vi "TagDB Refmgr-Parse Rules.vi"(0 "DB Ref":T3, 5 "Rules":T1[](array[typedef]), 11 "error in (no error)":errorcluster) -> (4 "DB Ref (dup)":T3, 6 "StateNames":string[](array[string]), 10 "RulesMap":variant[](array[variant]), 15 "error out":errorcluster)   [LabVIEW 2017, in "TagDB RefManager.lvlib"]
uses:
  TagDB RefManager.lvlib
  <userlib>/_NEVSTOP/TagDB/Typedef/TagDB.ctl
  Typedef/RefMgr-Logic-State.ctl
  Typedef/RefMgr-StateChangeType.ctl
  ad0d2cce-a5b7-4b1b-8c86-61dd78e8b0b8.vi
  <userlib>/_NEVSTOP/TagDB/TagDB.lvlib
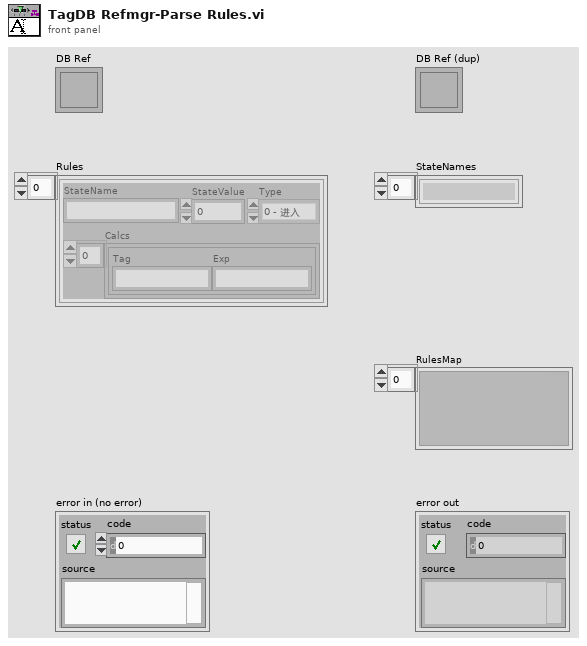
[diagram p1: front panel]
types:
  T1 = typedef "TagDB RefManager.lvlib/RefMgr-Logic-State.ctl" = cluster{"StateName":string, "StateValue":i32, "Type":T2, "Calcs":cluster{"Tag":string, "Exp":string}[]}
  T2 = typedef "TagDB RefManager.lvlib/RefMgr-StateChangeType.ctl" = enum16{"0 - 进入", "1 - 等于", "2 - 退出"}
  T3 = typedef "TagDB.lvlib/TagDB.ctl" = refnum<k1>
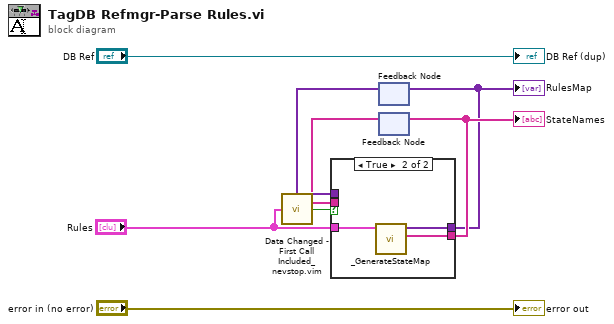
[diagram p0: block diagram]
diagram:
  n1 = call "Data Changed - First Call Included_nevstop.vim"("Variant"="Rules") -> ("Changed"=w4:bool)
  n2 = feedback #1() -> (w3:variant[])  [unwired: 1 in]
  n3 = feedback #2() -> (w2:string[])  [unwired: 1 in]
  n4 = case shown="True" w4 {
    tunnel: [w9 w13] -> w5
    tunnel: [w10 w12] -> w6
    tunnel: "Rules" -> [_ w11]
    tunnel: w3 -> [w9 _]
    tunnel: w2 -> [w10 _]
    frame False {
    }
    frame True {
      n5 = call "_GenerateStateMap.vi"("Rules"=w11) -> ("StateNames"=w12:string[], "RulesMap"=w13:variant[])  [unwired: 8 in, 1 out]
    }
  }
  "StateNames" <- w6
  "RulesMap" <- w5
  n6 = feedback-in #1(w5) -> ()
  n7 = feedback-in #2(w6) -> ()
  "error out" <- "error in (no error)"
  "DB Ref (dup)" <- "DB Ref"
